vi "Read Setting.vi"(8 "error in (no error)":errorcluster, 11 "Update DBL Array in":refnum<class "Update DBL Array.lvclass">) -> (0 "error out":errorcluster, 2 "Setting":dbl[](array[numeric]), 3 "Update DBL Array out":refnum<class "Update DBL Array.lvclass">)   [LabVIEW 2014, in "Update DBL Array.lvclass"]
uses:
  Update DBL Array.lvclass
  Update DBL Array.lvclass/Update DBL Array.ctl
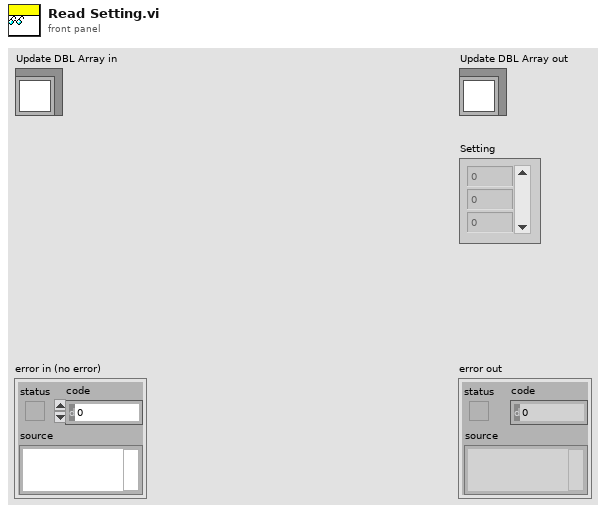
[diagram p1: front panel]
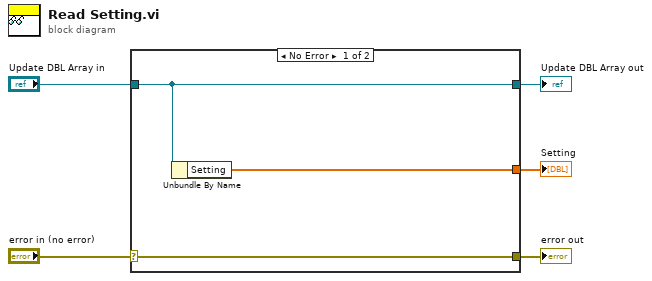
[diagram p0: block diagram]
diagram:
  n1 = case shown="No Error" "error in (no error)" {
    selector: "error in (no error)" -> [w8 w9]
    tunnel: [w8 w9] -> w4
    tunnel: [w7 w10] -> w2
    tunnel: "Update DBL Array in" -> [w7 w10]
    tunnel: [w6 _] -> w1
    frame No Error {
      n2 = Unbundle By Name(w7) -> ("Setting"=w6:dbl[])
    }
    frame Error {
    }
  }
  "error out" <- w4
  "Update DBL Array out" <- w2
  "Setting" <- w1
